vi "RT_Main.vi"() -> ()   [LabVIEW 2017]
uses:
  <vilib>/rvi/interface/nirviOpenFPGA/nirviOpenFPGA.xnode
  <vilib>/rvi/interface/nirviMethod/nirviMethod.xnode
  <vilib>/rvi/interface/nirviReadWriteControl/nirviReadWriteControl.xnode
  <vilib>/rvi/interface/nirviCloseFPGA/nirviCloseFPGA.xnode
  <vilib>/Utility/error.llb/Error Cluster From Error Code.vi
  <vilib>/rvi/interface/Simulation/niFpgaSimulationCallBeginRW.vi
  <vilib>/rvi/errors/niLvFpgaAdjustHostInterfaceError.vi
  NiFpgaLv.dll
  <vilib>/FPGAPlugInAG/Dynamic/niLvFpga_ConfigureFifo_Dynamic.vi
  <vilib>/rvi/errors/niLvFpgaMergeErrorWithErrorCode.vi
  <vilib>/FPGAPlugInAG/Dynamic/niLvFpga_StartFifo_Dynamic.vi
  <vilib>/FPGAPlugInAG/Dynamic/niLvFpga_Run_Dynamic.vi
  <vilib>/FPGAPlugInAG/Dynamic/niLvFpga_ReadFifo_Dynamic.vi
  <vilib>/FPGAPlugInAG/Dynamic/niLvFpga_Reset_Dynamic.vi
  <vilib>/Platform/TimedLoop/XDataNode/XDataNode.xnode
  <vilib>/Platform/TimedLoop/XDataNode/nitl_modes.ctl
  <vilib>/Platform/TimedLoop/XDataNode/XDNodeRunTimeDep.lvlib
  <vilib>/Platform/TimedLoop/XDataNode/wakeup.ctl
  <vilib>/Platform/TimedLoop/XDataNode/timing_clust.ctl
  <vilib>/Analysis/NI_AALBase.lvlib
  <vilib>/Analysis/baseanly.llb/Quick Scale 1D.vi
  <vilib>/FPGAPlugInAG/Dynamic/niLvFpga_Close_Dynamic.vi
  FPGA Bitfiles/MicrophoneArray_FPGATarget_fpga_U83CzskWL4Q.lvbitx
  FPGA_Main.vi
  <vilib>/FPGAPlugInAG/sbRIO-9636/niLvFpga_Open_sbRIO-9636.vi
  <vilib>/rvi/interface/common/dynamic/niFpgaDynamicAddResources.vi
panel:
  out "error out":errorcluster
  in  "error in":errorcluster
  out "Average Angle":dbl
  in  "Delay Multiplier":dbl=1.73
  out "Angles":dbl[](array[numeric])
  out "Sample Delay":dbl[](array[numeric])
  out "Mic 3 & 4 TDOA":dbl[](graph)
  out "Mic 2 & 3 TDOA":dbl[](graph)
  out "Mic 1 & 2 TDOA":dbl[](graph)
  out "Mic1_FIFO Timed Out?":bool
  out "Mic2_FIFO Timed Out?":bool
  out "Mic3_FIFO Timed Out?":bool
  out "Mic4 FIFO Timed Out?":bool
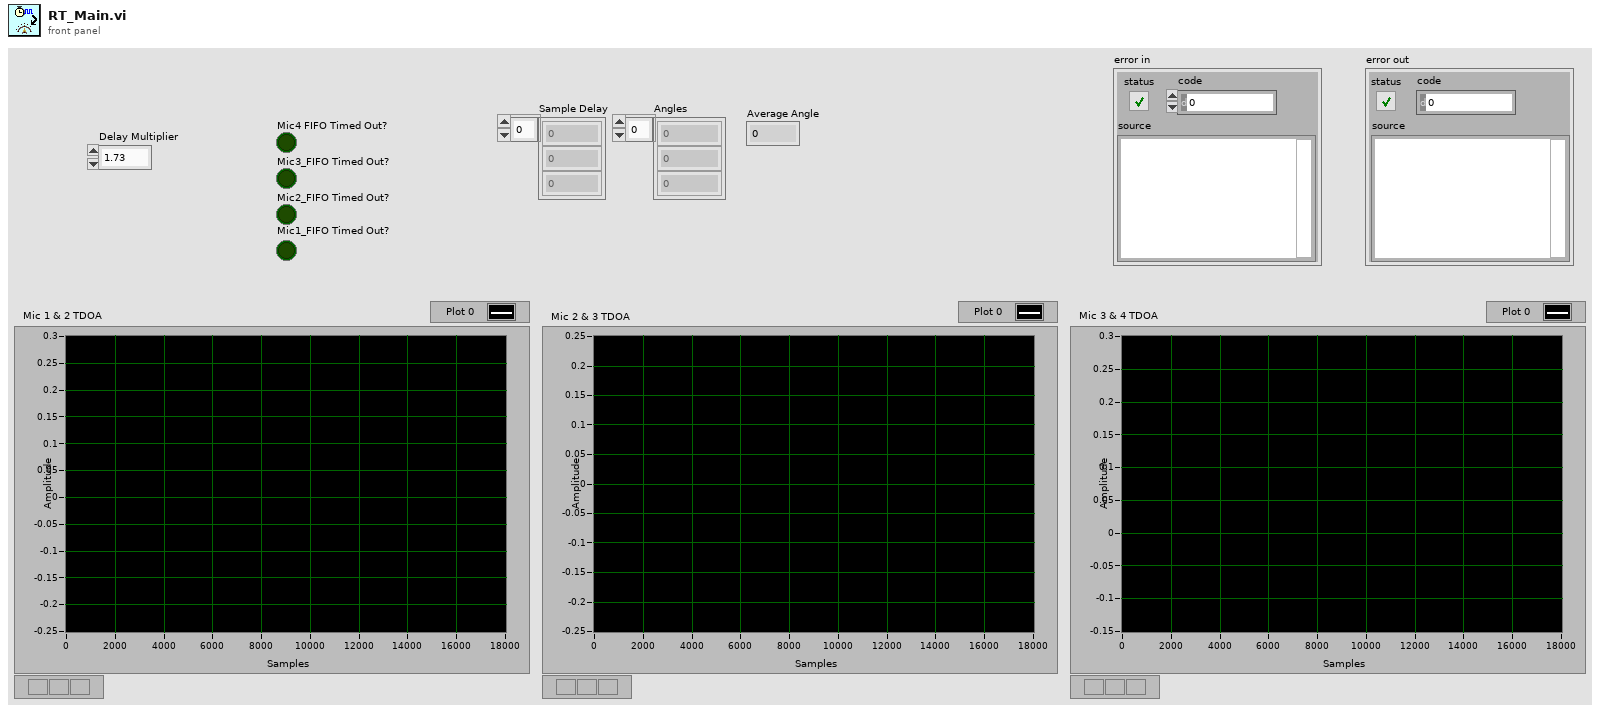
[diagram p1: front panel]
types:
  T1 = typedef "XDNodeRunTimeDep.lvlib/timing_clust.ctl" = cluster{"Expected End [f-1]":u64, "Actual End [f-1]":u64, "Finished Late? [f-1]":bool, "Expected End [i-1]":u64, "Actual End [i-1]":u64, "Finished Late? [i-1]":bool, "Expected Start [i]":u64, "Actual Start [i]":u64, "Expected Start [f]":u64, "Actual Start [f]":u64, "Source Name":string, "Structure Name":string, "Period":i64, "Deadline":i64, "Offset":i64, "Start":i64, "Priority":i32, "Timeout":i32, "Mode":T2, "Wakeup Reason":T3, "Error":errorcluster, "Source Type":string, "Secondary Source Type":string, "Global End Time":u64, "Global Start Time":u64, "Frame Duration":u64, "Iteration Duration":u64, "Assigned CPU":i32, "I/O Scan Engine Mode":u32}
  T2 = typedef "XDNodeRunTimeDep.lvlib/nitl_modes.ctl" = enum32{"No Change", "Process missed periods, maintain original phase", "Discard missed periods, maintain original phase", "Process missed periods, ignore original phase", "Discard missed periods, ignore original phase"}
  T3 = typedef "XDNodeRunTimeDep.lvlib/wakeup.ctl" = enum32{"Normal", "Aborted", "Asynchronous wakeup", "Timing source error", "Timed loop error", "Timeout"}
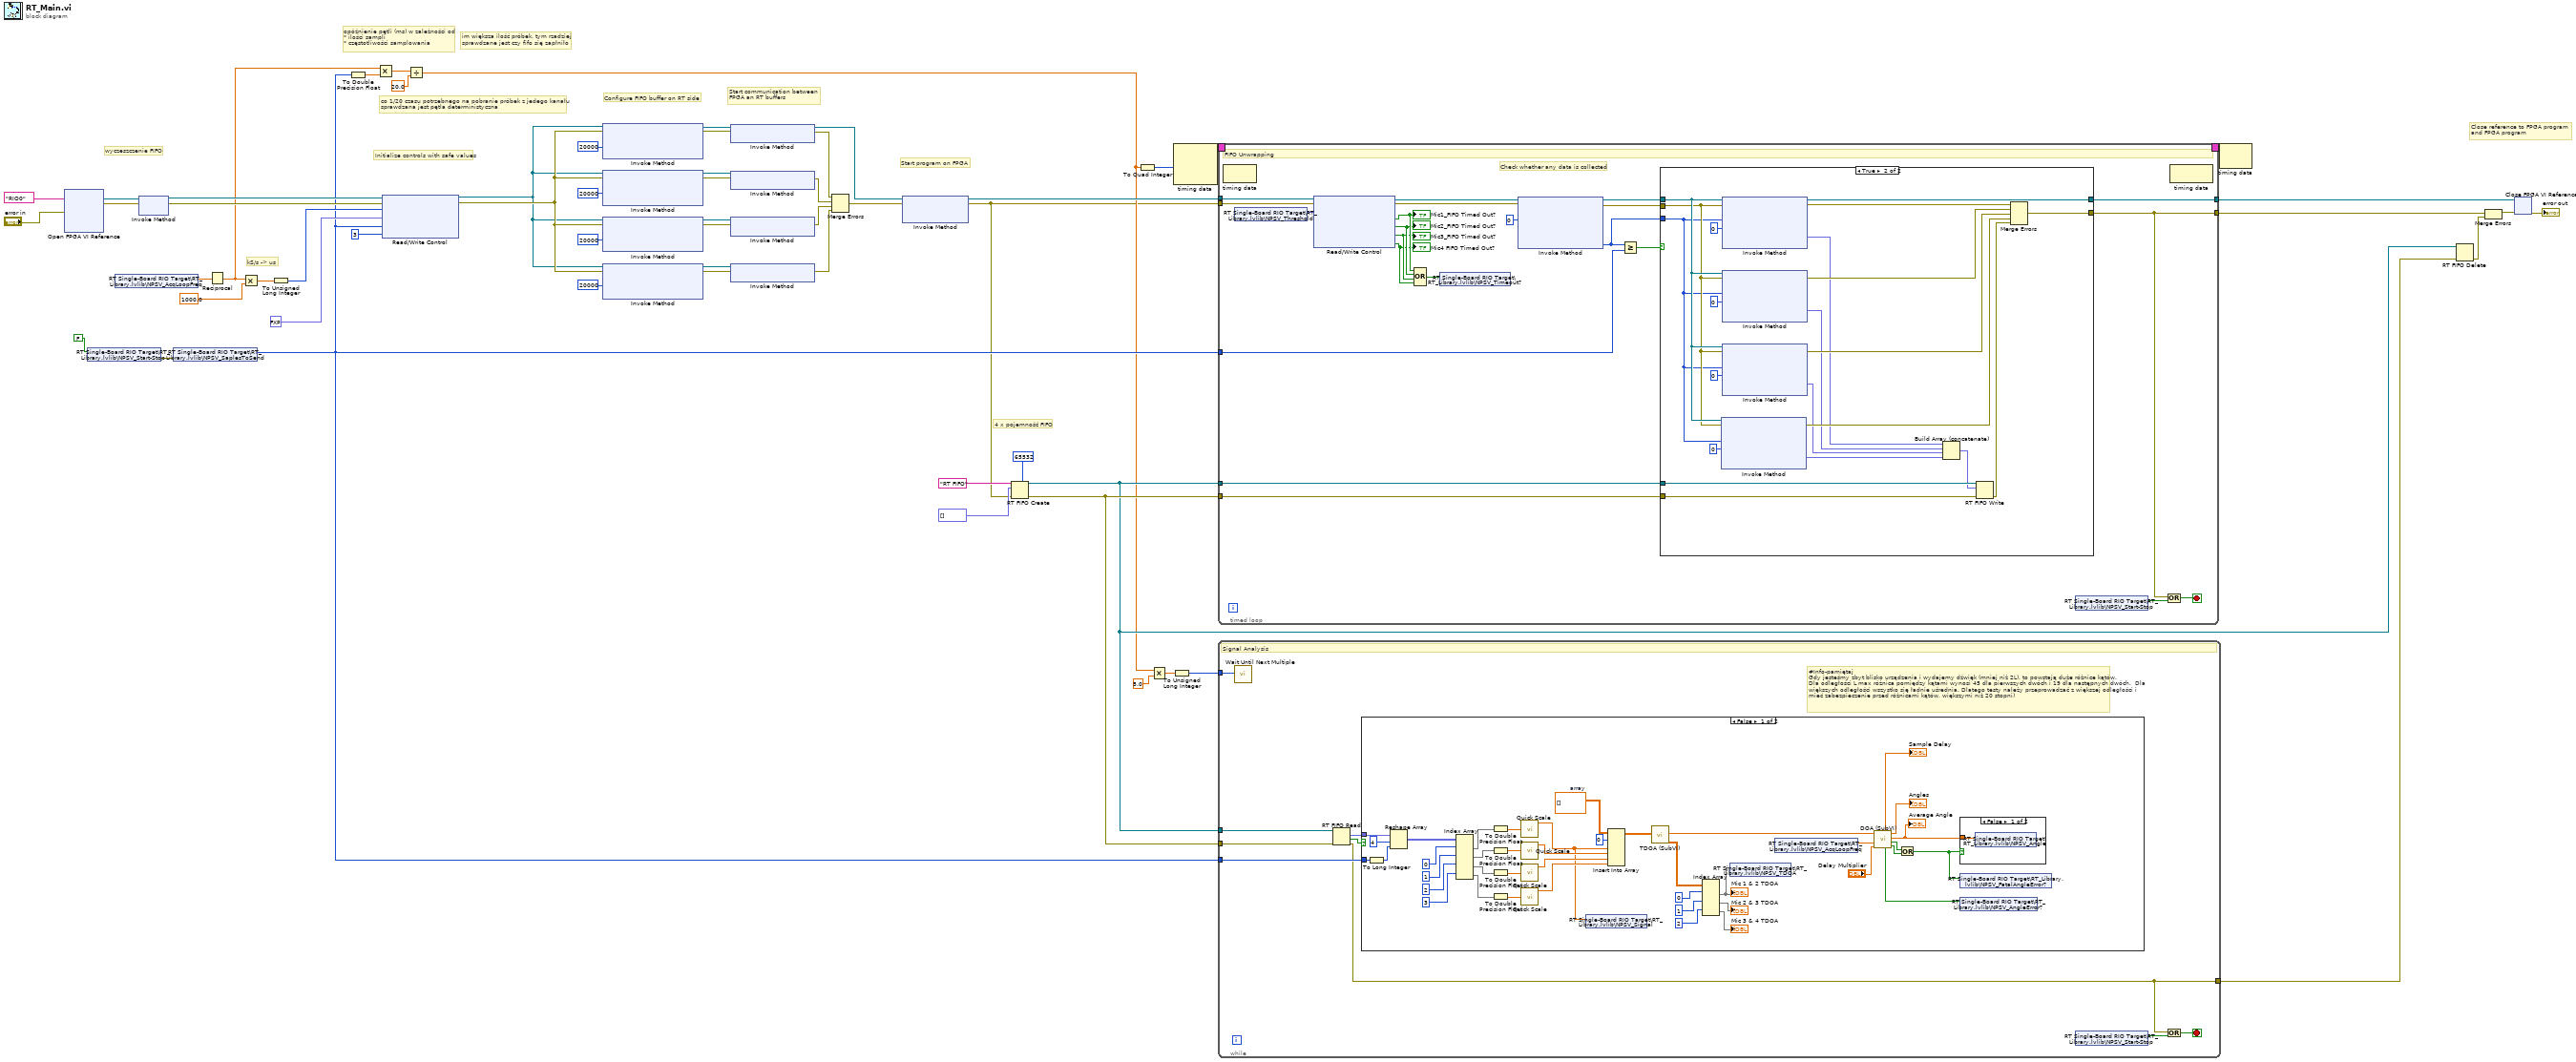
[diagram p0: block diagram]
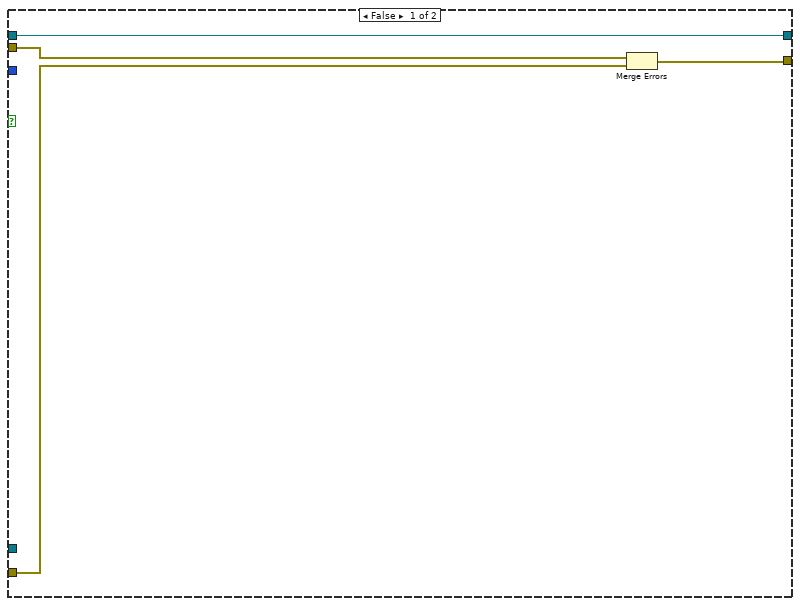
[diagram p2: hidden frame]
diagram:
  # "im większa ilość próbek, tym rzadziej \nsprawdzane jest czy fifo się zapłniło"
  # "co 1/20 czasu potrzebnego na pobranie próbek z jedego kanału \nsprawdzana jest pętla deterministyczna"
  # "opóźnienie pętli (ms) w zależności od \n* ilości sampli\n* częstotliwości samplowania"
  # "4 x pojemność FIFO"
  # "kS/s -> us"
  # "wyczeszczenie FIFO"
  # "Close reference to FPGA program \nand FPGA program"
  # "Start program on FPGA"
  # "Start communication between \nFPGA an RT buffers"
  # "Configure FIFO buffer on RT side"
  # "Initialize controls with safe values"
  n1 = xnode "Open FPGA VI Reference"("error in"="error in", "resource name"=tag "RIO0") -> ("FPGA VI Reference Out"=w31:refnum<k20>, "error out"=w39:errorcluster)
  n2 = shared-variable "RT Single-Board RIO Target\\RT_Library.lvlib\\NPSV_Start-Stop"(FALSE ("NPSV_Start-Stop")) -> (error out=w15:errorcluster)  [unwired: 1 in]
  n3 = shared-variable "RT Single-Board RIO Target\\RT_Library.lvlib\\NPSV_AcqLoopFreq"() -> (w14:dbl)  [unwired: 1 in, 1 out]
  n4 = xnode "Invoke Method"("FPGA VI Reference In"=w31, "error in"=w39) -> ("FPGA VI Reference Out"=w37:refnum<k20>, "error out"=w38:errorcluster)
  n5 = shared-variable "RT Single-Board RIO Target\\RT_Library.lvlib\\NPSV_SaplesToSend"(error in=w15) -> (w12:u32)  [unwired: 1 out]
  n6 = Reciprocal(x=w14) -> (1/x=w7:dbl)
  n7 = Multiply(x=w7, y=1000.0) -> (x*y=w30:dbl)
  n8 = To Unsigned Long Integer(number=w30) -> (unsigned 32bit integer=w29:u32)
  n9 = To Double Precision Float(number=w12) -> (double precision float=w13:dbl)
  n10 = Multiply(x=w7, y=w13) -> (x*y=w11:dbl)
  n11 = xnode "Read/Write Control"("FPGA VI Reference In"=w37, "error in"=w38, "AcqLoopDelay(uSec)"=w29, "Threshold"=fxp<+/-,28,9> 0.0, "SamplesToSend"=w12, "NoiseSamplesToReject"=u32 3) -> ("FPGA VI Reference Out"=w40:refnum<k20>, "error out"=w58:errorcluster)
  n12 = Divide(x=w11, y=20.0) -> (x/y=w5:dbl)
  n13 = xnode "Invoke Method"("FPGA VI Reference In"=w40, "error in"=w58, "Requested Depth"=u32 20000) -> ("FPGA VI Reference Out"=w57:refnum<k20>, "error out"=w21:errorcluster)  [unwired: 1 out]
  n14 = xnode "Invoke Method"("FPGA VI Reference In"=w40, "error in"=w58, "Requested Depth"=u32 20000) -> ("FPGA VI Reference Out"=w56:refnum<k20>, "error out"=w20:errorcluster)  [unwired: 1 out]
  n15 = xnode "Invoke Method"("FPGA VI Reference In"=w40, "error in"=w58, "Requested Depth"=u32 20000) -> ("FPGA VI Reference Out"=w55:refnum<k20>, "error out"=w19:errorcluster)  [unwired: 1 out]
  n16 = xnode "Invoke Method"("FPGA VI Reference In"=w40, "error in"=w58, "Requested Depth"=u32 20000) -> ("FPGA VI Reference Out"=w54:refnum<k20>, "error out"=w18:errorcluster)  [unwired: 1 out]
  n17 = xnode "Invoke Method"("FPGA VI Reference In"=w57, "error in"=w21) -> ("FPGA VI Reference Out"=w41:refnum<k20>, "error out"=w53:errorcluster)
  n18 = xnode "Invoke Method"("FPGA VI Reference In"=w56, "error in"=w20) -> ("error out"=w52:errorcluster)  [unwired: 1 out]
  n19 = xnode "Invoke Method"("FPGA VI Reference In"=w55, "error in"=w19) -> ("error out"=w51:errorcluster)  [unwired: 1 out]
  n20 = xnode "Invoke Method"("FPGA VI Reference In"=w54, "error in"=w18) -> ("error out"=w50:errorcluster)  [unwired: 1 out]
  n21 = Merge Errors(w53, w52, w51, w50) -> (w49:errorcluster)
  n22 = xnode "Invoke Method"("FPGA VI Reference In"=w41, "error in"=w49) -> ("FPGA VI Reference Out"=w48:refnum<k20>, "error out"=w1:errorcluster)  [unwired: 1 in]
  n23 = RT FIFO Create(0:"RT FIFO" ("name (unnamed)"), 1:fxp<+/-,28,9>[] [], 3:w1, 6:u32 65532 ("elements in array (1)")) -> (8:w25:refnum<k33>, 11:w26:errorcluster)  [unwired: 4 in, 1 out]
  n24 = To Quad Integer(1:w5) -> (0:w9:i64)
  n25 = Multiply(x=w5, y=5.0) -> (x*y=w6:dbl)
  n26 = node-c288(w9) -> (w35:T1)  [unwired: 2 in]
  n27 = To Unsigned Long Integer(number=w6) -> (unsigned 32bit integer=w8:u32)
  n28 = timed-loop {
    tunnel: w48 -> [w81]
    tunnel: w1 -> [w80]
    tunnel: [w76] -> w47
    tunnel: [w60] -> w22
    tunnel: w12 -> [w72]
    timing: w35 -> [_]
    timing-out: [_] -> w34
    tunnel: w25 -> [w70]
    tunnel: w26 -> [w69]
    stop <- w61 stop-if-true
    # "Check whether any data is collected"
    # "FIFO Unwrapping"
    n29 = node-c288() -> ()  [unwired: 1 in, 1 out]
    n30 = shared-variable "RT Single-Board RIO Target\\RT_Library.lvlib\\NPSV_Threshold"() -> (w63:fxp<+/-,28,9>)  [unwired: 1 in, 1 out]
    n31 = xnode "Read/Write Control"("FPGA VI Reference In"=w81, "error in"=w80, "Threshold"=w63) -> ("FPGA VI Reference Out"=w73:refnum<k20>, "error out"=w74:errorcluster, "Mic_1_FIFO_Timed Out?"=w68:bool, "Mic_2_FIFO_Timed Out?"=w67:bool, "Mic_3_FIFO_Timed Out?"=w66:bool, "Mic_4_FIFO_Timed Out?"=w65:bool)
    "Mic4 FIFO Timed Out?" <- w65
    "Mic3_FIFO Timed Out?" <- w66
    "Mic2_FIFO Timed Out?" <- w67
    "Mic1_FIFO Timed Out?" <- w68
    n32 = Compound Arithmetic op=OR(w68, w67, w66, w65) -> (w64:bool)
    n33 = shared-variable "RT Single-Board RIO Target\\RT_Library.lvlib\\NPSV_Timeout?"(w64) -> ()  [unwired: 1 in, 1 out]
    n34 = xnode "Invoke Method"("FPGA VI Reference In"=w73, "error in"=w74, "Number of Elements"=u32 0) -> ("FPGA VI Reference Out"=w78:refnum<k20>, "error out"=w77:errorcluster, "Elements Remaining"=w75:u32)  [unwired: 1 in, 1 out]
    n35 = Greater Or Equal?(x=w75, y=w72) -> (x >= y?=w71:bool)
    n36 = case shown="True" w71 {
      tunnel: w78 -> [w87 w108]
      tunnel: w77 -> [w85 w107]
      tunnel: [w87 w102] -> w76
      tunnel: [w86 w101] -> w60
      tunnel: w75 -> [_ w89]
      tunnel: w70 -> [_ w92]
      tunnel: w69 -> [w84 w91]
      frame False {
        n37 = Merge Errors(w85, w84) -> (w86:errorcluster)
      }
      frame True {
        n38 = xnode "Invoke Method"("FPGA VI Reference In"=w108, "error in"=w107, "Number of Elements"=w89, "Timeout (ms)"=0) -> ("error out"=w103:errorcluster, "Data"=w94:fxp<+/-,28,9>[])  [unwired: 2 out]
        n39 = xnode "Invoke Method"("FPGA VI Reference In"=w108, "error in"=w107, "Number of Elements"=w89, "Timeout (ms)"=0) -> ("FPGA VI Reference Out"=w102:refnum<k20>, "error out"=w106:errorcluster, "Data"=w96:fxp<+/-,28,9>[])  [unwired: 1 out]
        n40 = xnode "Invoke Method"("FPGA VI Reference In"=w108, "error in"=w107, "Number of Elements"=w89, "Timeout (ms)"=0) -> ("error out"=w105:errorcluster, "Data"=w95:fxp<+/-,28,9>[])  [unwired: 2 out]
        n41 = xnode "Invoke Method"("FPGA VI Reference In"=w108, "error in"=w107, "Number of Elements"=w89, "Timeout (ms)"=0) -> ("error out"=w104:errorcluster, "Data"=w93:fxp<+/-,28,9>[])  [unwired: 2 out]
        n42 = Build Array (concatenate)(w96, w95, w93, w94) -> (w88:fxp<+/-,28,9>[])
        n43 = RT FIFO Write(0:w92, 1:w88, 3:w91) -> (11:w90:errorcluster)  [unwired: 2 in, 3 out]
        n44 = Merge Errors(w106, w105, w104, w103, w90) -> (w101:errorcluster)
      }
    }
    n45 = shared-variable "RT Single-Board RIO Target\\RT_Library.lvlib\\NPSV_Start-Stop"() -> (w62:bool)  [unwired: 1 in, 1 out]
    n46 = Or(x=w60, y=w62) -> (x .or. y?=w61:bool)
    n47 = node-c288() -> ()  [unwired: 1 in, 1 out]
  }
  n48 = while {
    tunnel: w25 -> [w117]
    tunnel: w26 -> [w116]
    tunnel: [w109] -> w17
    tunnel: w12 -> [w115]
    tunnel: w8 -> [w112]
    stop <- w111 stop-if-true
    # "#Info-pamiętaj\nGdy jesteśmy zbyt blisko urządzenia i wydajemy dźwięk (mniej niż 2L), to powstają duże różnice kątów.\nDla odległości L max różnica pomiędzy kątami wynosi 45 dla pierwszych dwóch i 19 dla następnych dwóch.  Dla większych odległości wszystko się ładnie uśrednia. Dlatego testy należy przeprowadzać z większej odległości i mieć zabezpieczenie przed różnicami kątów, większymi niż 20 stopni)"
    # "Signal Analysis"
    n49 = call "Wait Until Next Multiple"("Count(mSec)"=w112) -> ()  [unwired: 1 out]
    n50 = RT FIFO Read(0:w117, 3:w116) -> (9:w114:fxp<+/-,28,9>[], 10:w113:bool, 11:w109:errorcluster)  [unwired: 2 in, 2 out]
    n51 = case shown="False" w113 {
      tunnel: w115 -> [w158 _]
      tunnel: w114 -> [w157 _]
      frame False {
        w150 = dbl[][] []  # array
        n52 = To Long Integer(number=w158) -> (32bit integer=w137:i32)
        n53 = Reshape Array(w157, 4 ("dimension size"), w137) -> (w155:fxp<+/-,28,9>[][])
        n54 = Index Array(array=w155, index (row) #1=0 ("index (row)"), index (row) #2=1 ("index (row)"), index (row) #3=2 ("index (row)"), index (row) #4=3 ("index (row)")) -> (element #1=w130:fxp<+/-,28,9>[], element #2=w132:fxp<+/-,28,9>[], element #3=w134:fxp<+/-,28,9>[], element #4=w135:fxp<+/-,28,9>[])  [unwired: 4 in]
        n55 = To Double Precision Float(number=w130) -> (double precision float=w129:dbl[])
        n56 = To Double Precision Float(number=w132) -> (double precision float=w131:dbl[])
        n57 = To Double Precision Float(number=w134) -> (double precision float=w133:dbl[])
        n58 = To Double Precision Float(number=w135) -> (double precision float=w136:dbl[])
        n59 = call-poly <vilib>:"Quick Scale.vi"("X"=w129) -> ("Y[i]=X[i]/Max|X|"=w119:dbl[])  [unwired: 2 out]
        n60 = call-poly <vilib>:"Quick Scale.vi"("X"=w131) -> ("Y[i]=X[i]/Max|X|"=w139:dbl[])  [unwired: 2 out]
        n61 = call-poly <vilib>:"Quick Scale.vi"("X"=w133) -> ("Y[i]=X[i]/Max|X|"=w140:dbl[])  [unwired: 2 out]
        n62 = call-poly <vilib>:"Quick Scale.vi"("X"=w136) -> ("Y[i]=X[i]/Max|X|"=w141:dbl[])  [unwired: 2 out]
        n63 = shared-variable "RT Single-Board RIO Target\\RT_Library.lvlib\\NPSV_Signal"(w119) -> ()  [unwired: 1 in, 1 out]
        n64 = Insert Into Array(array=w150, index (row)=0, new element #1=w119, new element #2=w139, new element #3=w140, new element #4=w141) -> (w148:dbl[][])  [unwired: 1 in]
        n65 = call "TDOA (SubVI).vi"("signal array"=w148) -> ("tdoa arrays"=w144:dbl[][], "delay array"=w138:dbl[])  [unwired: 9 in]
        n66 = Index Array(array=w144, index (row) #1=0 ("index (row)"), index (row) #2=1 ("index (row)"), index (row) #3=2 ("index (row)")) -> (element #1=w120:dbl[], element #2=→"Mic 2 & 3 TDOA":dbl[], element #3=→"Mic 3 & 4 TDOA":dbl[])  [unwired: 3 in]
        "Mic 1 & 2 TDOA" <- w120
        n67 = shared-variable "RT Single-Board RIO Target\\RT_Library.lvlib\\NPSV_TDOA"(w120) -> ()  [unwired: 1 in, 1 out]
        n68 = shared-variable "RT Single-Board RIO Target\\RT_Library.lvlib\\NPSV_AcqLoopFreq"() -> (w128:dbl)  [unwired: 1 in, 1 out]
        n69 = call "DOA (SubVI).vi"("fix delay"="Delay Multiplier", "sampling freq"=w128, "delay array"=w138) -> ("fatal angle error?"=w124:bool, "NaN?"=w125:bool, "average angle"=w121:dbl, "angles"=→"Angles":dbl[], "angle error?"=w123:bool, "sample delay"=→"Sample Delay":dbl[])  [unwired: 3 in]
        "Average Angle" <- w121
        n70 = Or(x=w125, y=w124) -> (x .or. y?=w122:bool)
        n71 = case shown="False" w122 {
          tunnel: w121 -> [w159 _]
          frame False {
            n72 = shared-variable "RT Single-Board RIO Target\\RT_Library.lvlib\\NPSV_Angle"(w159) -> ()  [unwired: 1 in, 1 out]
          }
          frame True {
          }
        }
        n73 = shared-variable "RT Single-Board RIO Target\\RT_Library.lvlib\\NPSV_FatalAngleError?"(w122) -> ()  [unwired: 1 in, 1 out]
        n74 = shared-variable "RT Single-Board RIO Target\\RT_Library.lvlib\\NPSV_AngleError?"(w123) -> ()  [unwired: 1 in, 1 out]
      }
      frame True {
      }
    }
    n75 = shared-variable "RT Single-Board RIO Target\\RT_Library.lvlib\\NPSV_Start-Stop"() -> (w110:bool)  [unwired: 1 in, 1 out]
    n76 = Or(x=w109, y=w110) -> (x .or. y?=w111:bool)
  }
  n77 = node-c288(w34) -> ()  [unwired: 1 out]
  n78 = RT FIFO Delete(0:w25, 3:w17) -> (11:w23:errorcluster)  [unwired: 1 in]
  n79 = Merge Errors(w22, w23) -> (w24:errorcluster)
  n80 = xnode "Close FPGA VI Reference"("FPGA VI Reference In"=w47, "error in"=w24) -> ("error out"=→"error out":errorcluster)
